vi "FTW-SQLite-Backup.vi"(0 "SQLite Connection":refnum<data-value>, 5 "Destination Database Filepath":path, 11 "error in":errorcluster) -> (4 "SQLite Connection out":refnum<data-value>, 6 "Time to Execute":dbl format="%.6fsec", 15 "error out":errorcluster)   [LabVIEW 2015]
uses:
  core/FTW-SQLite-Core-Structure.ctl
  core/FTW-SQLite-Core-AccessMode.ctl
panel:
  # "Inputs"
  # "Outputs"
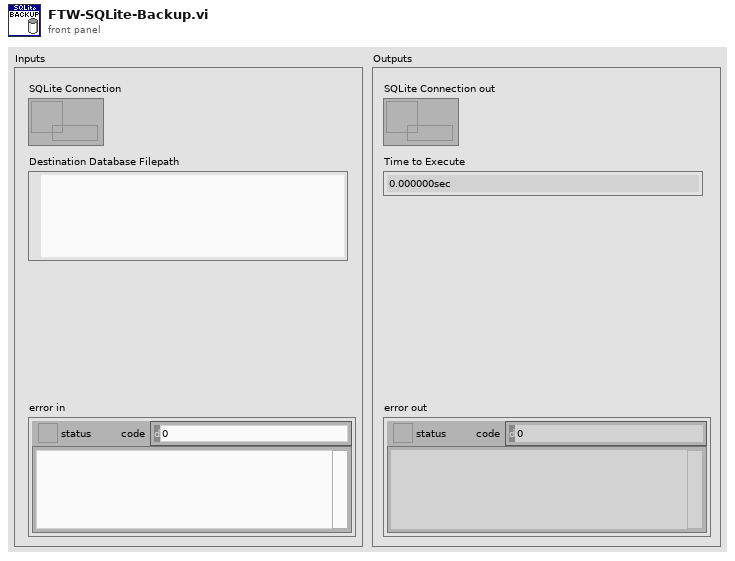
[diagram p1: front panel]
types:
  T1 = typedef "FTW-SQLite-Core-AccessMode.ctl" = enum16{"Read", "Read/Write", "Read/Write/Create"}
  T2 = typedef "FTW-SQLite-Core-Structure.ctl" = cluster{"Connection":u64}
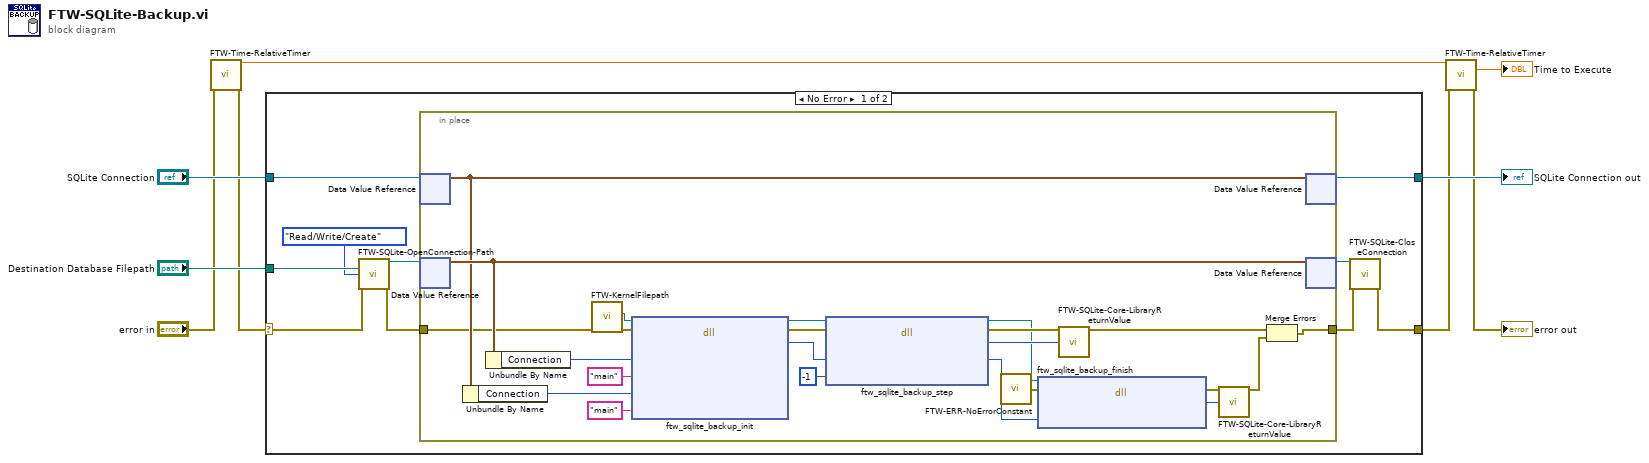
[diagram p0: block diagram]
diagram:
  n1 = call "FTW-Time-RelativeTimer.vi"("error in"="error in") -> ("Current Timer Value"=w4:dbl, "error out"=w5:errorcluster)  [unwired: 12 in, 1 out]
  n2 = case shown="No Error" w5 {
    selector: w5 -> [w18 w43]
    tunnel: "SQLite Connection" -> [w11 w44]
    tunnel: [w10 w44] -> w8
    tunnel: "Destination Database Filepath" -> [w19 _]
    tunnel: [w15 w43] -> w2
    frame No Error {
      n3 = call "FTW-SQLite-OpenConnection-Path.vi"("Database Filepath"=w19, "Access Mode"=FTW-SQLite-Core-AccessMode."Read/Write/Create", "error in"=w18) -> ("SQLite Connection"=w13:refnum<data-value>, "error out"=w17:errorcluster)  [unwired: 11 in]
      n4 = in-place {
        in-place-border: w17 -> [w24]
        in-place-border: [w29] -> w16
        n5 = in-place-dvr #1(w11) -> (w25:T2)  [unwired: 1 out]
        n6 = in-place-dvr #2(w13) -> (w28:T2)  [unwired: 1 out]
        n7 = Unbundle By Name(w25) -> ("Connection"=w26:u64)
        n8 = Unbundle By Name(w28) -> ("Connection"=w27:u64)
        n9 = call "FTW-KernelFilepath.vi"("error in"=w24) -> ("error out"=w23:errorcluster, "Library Filepath"=w22:path)  [unwired: 8 in, 1 out]
        n10 = dll-call lib="?" fn="ftw_sqlite_backup_init"(path in=w22, error in=w23, "Destination Pointer"=w27, "Destination Name"="main", "Source Pointer"=w26, "Source Name"="main") -> (path out=w21:path, error out=w31:errorcluster, "Backup Object"=w33:u64)  [unwired: 5 in]
        n11 = dll-call lib="?" fn="ftw_sqlite_backup_step"(path in=w21, error in=w31, "Backup Object"=w33, "NumPages"=-1) -> (path out=w20:path, error out=w36:errorcluster, "Return Type"=w34:i32, "Backup Object"=w42:u64)  [unwired: 2 in]
        n12 = call "FTW-ERR-NoErrorConstant.vi"() -> ("no error"=w32:errorcluster)
        n13 = dll-call lib="?" fn="ftw_sqlite_backup_finish"(path in=w20, error in=w32, "Backup Object"=w42) -> (error out=w41:errorcluster, "Return Value"=w40:i32)  [unwired: 2 in, 1 out]
        n14 = call "FTW-SQLite-Core-LibraryReturnValue.vi"("error in"=w36, "Return Value"=w34) -> ("error out"=w35:errorcluster)  [unwired: 13 in]
        n15 = call "FTW-SQLite-Core-LibraryReturnValue.vi"("error in"=w41, "Return Value"=w40) -> ("error out"=w39:errorcluster)  [unwired: 13 in]
        n16 = Merge Errors(w35, w39) -> (w29:errorcluster)
        n17 = in-place-dvr #1(w25) -> (w10:refnum<data-value>)  [unwired: 1 out]
        n18 = in-place-dvr #2(w28) -> (w12:refnum<data-value>)  [unwired: 1 out]
      }
      n19 = call "FTW-SQLite-CloseConnection.vi"("SQLite Connection"=w12, "error in"=w16) -> ("error out"=w15:errorcluster)  [unwired: 13 in]
    }
    frame Error {
    }
  }
  "SQLite Connection out" <- w8
  n20 = call "FTW-Time-RelativeTimer.vi"("Previous Timer Value"=w4, "error in"=w2) -> ("Elapsed Time"=→"Time to Execute":dbl, "error out"=→"error out":errorcluster)  [unwired: 11 in, 1 out]
